vi "Calculate Subroutine.vi"(8 "Max Cup":i32, 9 "Start Cup":i32, 10 "Start Array":i32[](array[numeric]), 11 "Moves":i32) -> (3 "End Array":i32[](array[numeric]))   [LabVIEW 2020]
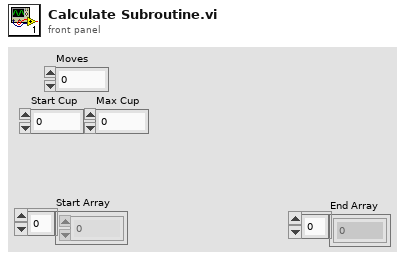
[diagram p1: front panel]
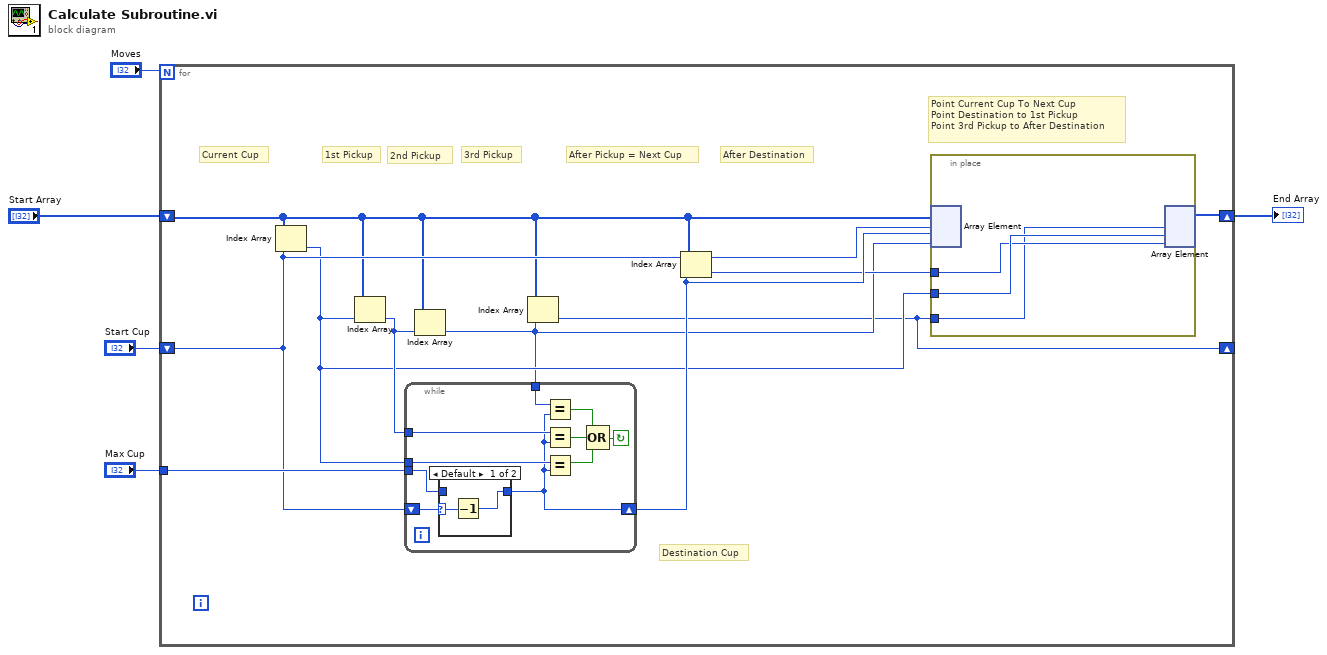
[diagram p0: block diagram]
diagram:
  n1 = for {
    N: "Moves" -> [_]
    shift-right: [w13] -> w5
    shift-left: "Start Array" -> [w8]
    shift-right: [w6] -> _
    shift-left: "Start Cup" -> [w12]
    tunnel: "Max Cup" -> [w14]
    # "After Destination"
    # "Point Current Cup To Next Cup\nPoint Destination to 1st Pickup\nPoint 3rd Pickup to After Destination"
    # "After Pickup = Next Cup"
    # "Destination Cup"
    # "3rd Pickup"
    # "2nd Pickup"
    # "1st Pickup"
    # "Current Cup"
    n2 = Index Array(array=w8, index=w12) -> (element=w9:i32)
    n3 = Index Array(array=w8, index=w9) -> (element=w15:i32)
    n4 = Index Array(array=w8, index=w15) -> (element=w7:i32)
    n5 = while {
      tunnel: w7 -> [w28]
      tunnel: w15 -> [w27]
      tunnel: w9 -> [w26]
      shift-right: [w19] -> w11
      shift-left: w12 -> [w21]
      tunnel: w14 -> [w20]
      stop <- w22 continue-if-true
      n6 = case shown="Default" w21 {
        selector: w21 -> [w30 _]
        tunnel: w20 -> [_ w31]
        tunnel: [w29 w31] -> w19
        frame Default {
          n7 = Decrement(x=w30) -> (x-1=w29:i32)
        }
        frame 1 {
        }
      }
      n8 = Equal?(x=w28, y=w19) -> (x = y?=w24:bool)
      n9 = Equal?(x=w27, y=w19) -> (x = y?=w25:bool)
      n10 = Equal?(x=w26, y=w19) -> (x = y?=w23:bool)
      n11 = Compound Arithmetic op=OR(w24, w25, w23) -> (w22:bool)
    }
    n12 = Index Array(array=w8, index=w7) -> (element=w6:i32)
    n13 = Index Array(array=w8, index=w11) -> (element=w10:i32)
    n14 = in-place {
      in-place-border: w9 -> [w18]
      in-place-border: w10 -> [w17]
      in-place-border: w6 -> [w16]
      n15 = in-place-array #1(w8, w12, w11, w7) -> ()  [unwired: 3 out]
      n16 = in-place-array #1(w16, w18, w17) -> (w13:i32[])  [unwired: 3 out]
    }
  }
  "End Array" <- w5
